vi "FPGA_8a_2ws_BIdireccional.vi"() -> ()   [LabVIEW 2015]
doc: "This VI reads a buffer of single point values from all four channels of the NI 923x and places the acquired data into a DMA FIFO."
uses:
  <vilib>/LabVIEW Targets/FPGA/cRIO/shared/nicrio_ModuleControls/nicrio_cRIO-9234_DataRatesRing2.ctl
  <vilib>/LabVIEW Targets/FPGA/cRIO/shared/nicrio_ModuleControls/nicrio_BasicConversionTime.ctl
  <vilib>/rvi/Emulation/niFpgaGetClockAttributes.vi
  <vilib>/rvi/Emulation/niFpgaSctlEmulationGetInTimedLoop.vi
  <vilib>/rvi/Emulation/niFpgaEmulationReportErrorSimple.vi
  <vilib>/rvi/Emulation/niFpgaProcessEmulError.vi
  <vilib>/rvi/eio/common/nirviEmuTemplateMethod_errors.vi
  <vilib>/rvi/Emulation/niFpgaCriticalErrorInLSC.vi
  <vilib>/rvi/eio/common/nirviEmuTemplatePropertySet_errors.vi
  <vilib>/rvi/interface/RandomDataEmulation/niFpgaRandomDataHandleErrors.vi
  <vilib>/eio/EIONode/EIONode.xnode
  <vilib>/eio/EIOPropertyNode/EIOPropertyNode.xnode
  <vilib>/rvi/DataTransferAndStorage/Container/XNode/niFpgaContainer.xnode
  <vilib>/rvi/interface/RandomDataEmulation/nirviRandomDataFpgaReadWriteTemplate.vi
  <vilib>/rvi/eio/common/nirviEmuTemplatePropertyGet_errors.vi
  <vilib>/rvi/eio/common/nirviEmuTemplatePropertyGet_noerrors.vi
  <vilib>/rvi/eio/common/nirviEmuTemplatePropertySet_noerrors.vi
panel:
  in  "Cycles to Filter":u16=5
  in  "Offset_WS2":fxp<+/-,24,-4>=0.000999998301267624 format="%.27g"
  in  "Canal cero WS2?":bool=TRUE
  out "NºRuedas 2":i32
  out "Nº Ruedas 1":i32
  out "Parar":bool
  out "RuedaDetectada2?":bool
  out "RuedaDetectada1?":bool
  out "Rueda2?":i16
  out "WhlCnt2":fxp<+/-,24,-4> format="%.27g"
  out "Direccion 0?":bool
  in  "Digital?":bool=TRUE
  out "Numeric 2":i32
  out "WhlCnt1":fxp<+/-,24,-4> format="%.27g"
  in  "Offset_WS1":fxp<+/-,24,-4>=0.000999998301267624 format="%.27g"
  out "Rueda1?":i16
  in  "Conversion Time":T1
  in  "Canal cero WS1?":bool=TRUE
  in  "Count(mSec)":u32=2
  out "Chassis Temperature":i16
  out "Detector de\npresencia":bool
  in  "Fotocélula":bool
  out "DC OK":bool
  in  "Data Rate":T2=2 items=["51.200 kS/s (NI 9234)"=1, "25.600 kS/s (NI 9234)"=2, "17.067 kS/s (NI 9234)"=3, "12.800 kS/s (NI 9234)"=4, "10.240 kS/s (NI 9234)"=5, "8.533 kS/s (NI 9234)"=6, "7.314 kS/s (NI 9234)"=7, "6.400 kS/s (NI 9234)"=8, "5.689 kS/s (NI 9234)"=9, "5.120 kS/s (NI 9234)"=10, "4.654 kS/s (NI 9234)"=11, "4.267 kS/s (NI 9234)"=12, "3.938 kS/s (NI 9234)"=13, "3.657 kS/s (NI 9234)"=14, "3.413 kS/s (NI 9234)"=15, "3.200 kS/s (NI 9234)"=16, "3.012 kS/s (NI 9234)"=17, "2.845 kS/s (NI 9234)"=18, "2.695 kS/s (NI 9234)"=19, "2.560 kS/s (NI 9234)"=20, "2.438 kS/s (NI 9234)"=21, "2.328 kS/s (NI 9234)"=22, "2.226 kS/s (NI 9234)"=23, "2.133 kS/s (NI 9234)"=24, "2.048 kS/s (NI 9234)"=25, "1.969 kS/s (NI 9234)"=26, "1.896 kS/s (NI 9234)"=27, "1.829 kS/s (NI 9234)"=28, "1.765 kS/s (NI 9234)"=29, "1.707 kS/s (NI 9234)"=30, "1.652 kS/s (NI 9234)"=31]
  out "Buffer Overflow":bool
  in  "Stop":bool
  out "Buffer Underflow":bool
  out "Error Out":errorcluster
  # "For instructions, and select Help>>Show Context Help and hover over the icon."
  # "Timing Parameters"
  # "Output Parameters"
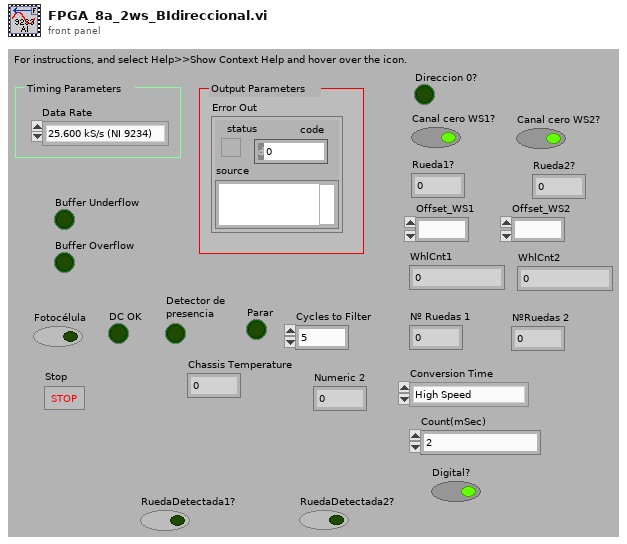
[diagram p1: front panel]
types:
  T1 = typedef "nicrio_BasicConversionTime.ctl" = enum8{"High Speed", "High Resolution"}
  T2 = typedef "nicrio_cRIO-9234_DataRatesRing2.ctl" = u8
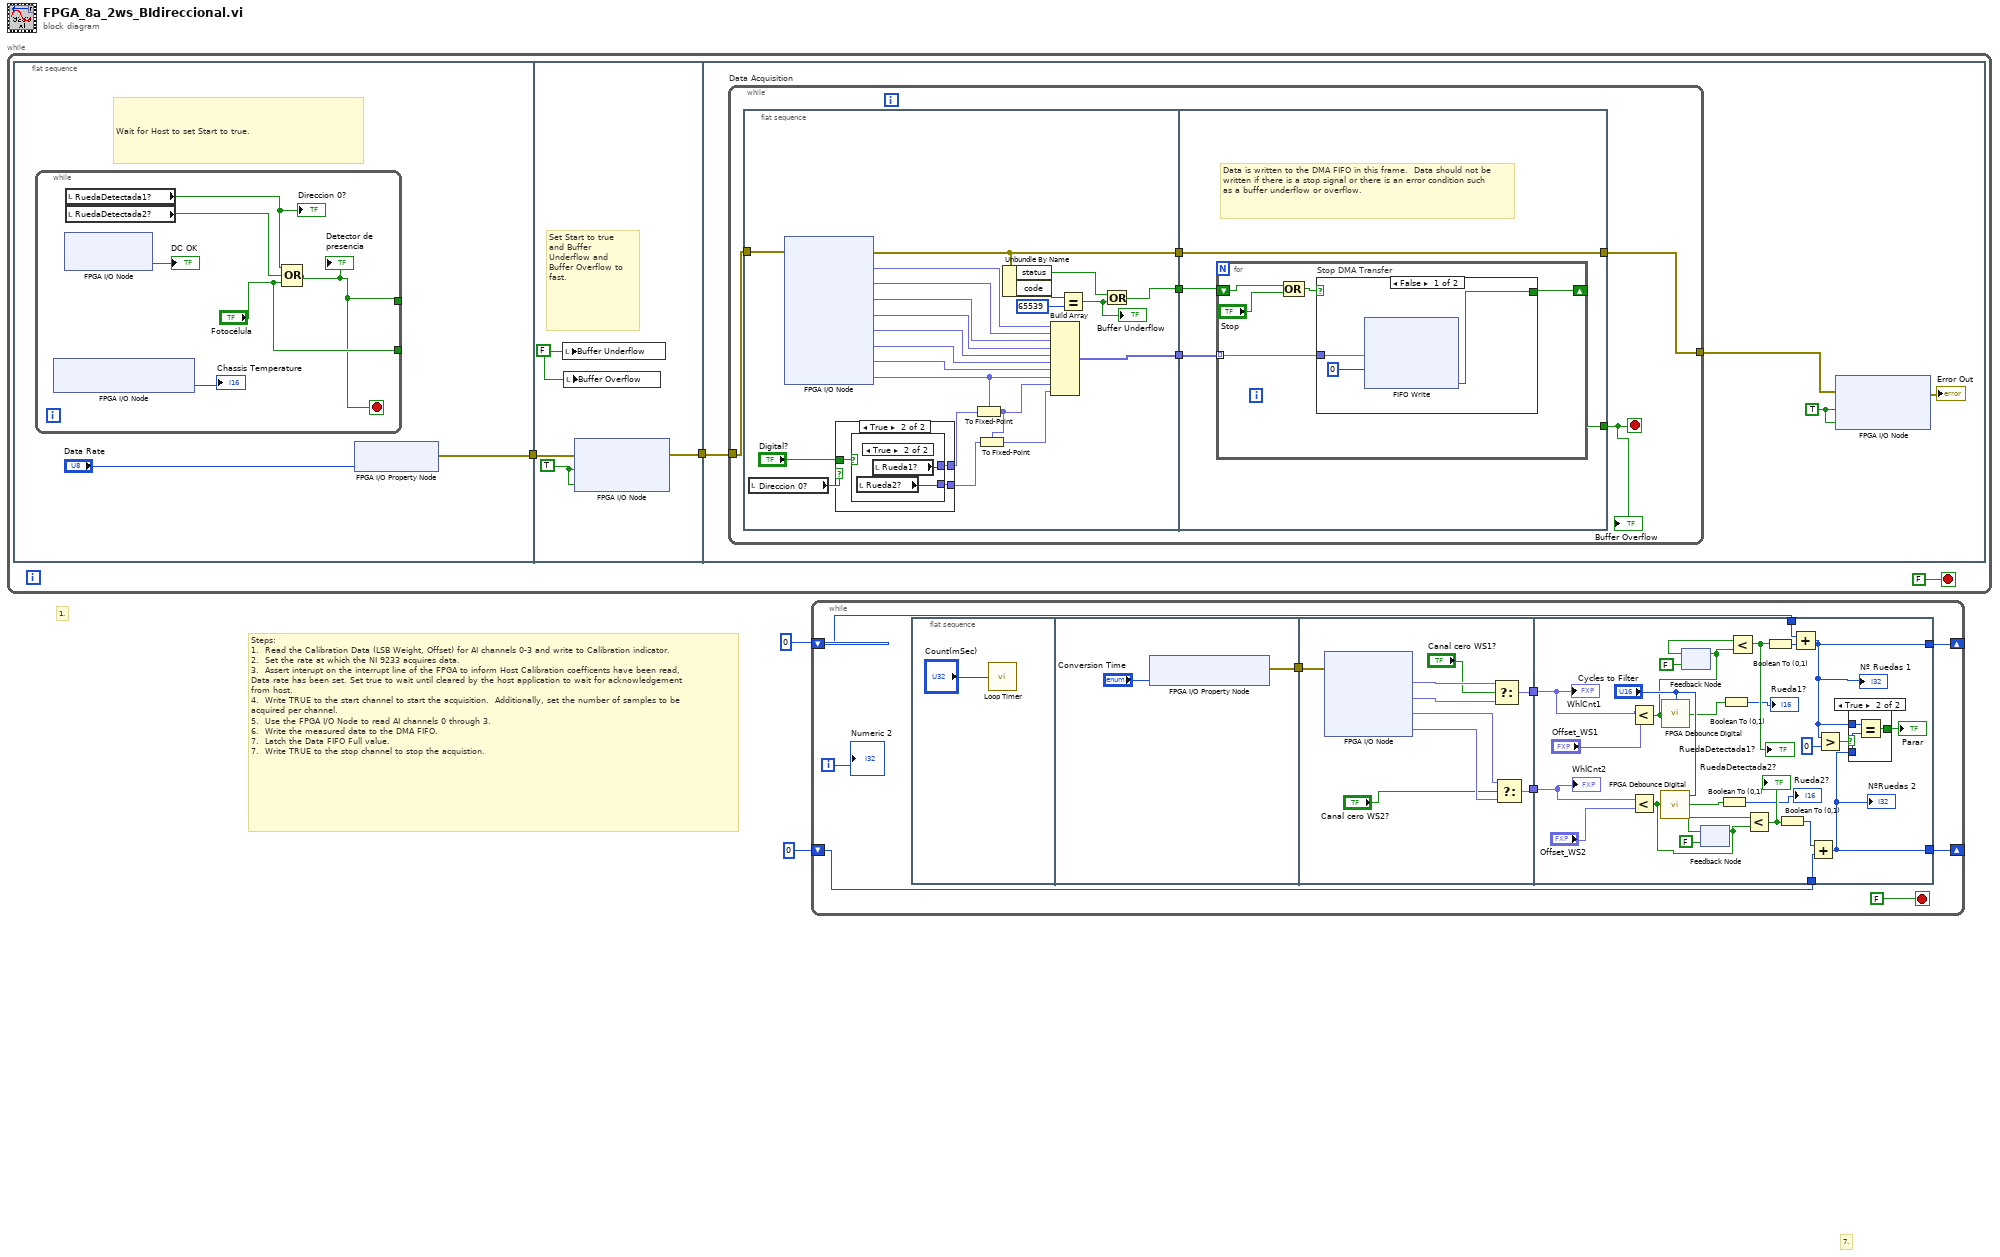
[diagram p0: block diagram]
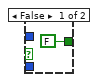
[diagram p2: hidden frame]
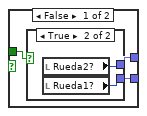
[diagram p3: hidden frame]
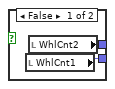
[diagram p4: hidden frame]
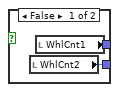
[diagram p5: hidden frame]
diagram:
  # "Steps: \n1.  Read the Calibration Data (LSB Weight, Offset) for AI channels 0-3 and write to Calibration indicator.\n2.  Set the rate at which the NI 9233 acquires data. \n3.  Assert interupt on the interrupt line of the FPGA to inform Host Calibration coefficents have been read, Data rate has been set. Set true to wait until cleared by the host application to wait for acknowledgement from host.\n4.  Write TRUE to the start channel to start the acquisition.  Additionally, set the number of samples to be acquired per channel.\n5.  Use the FPGA I/O Node to read AI channels 0 through 3. \n6.  Write the measured data to the DMA FIFO.\n7.  Latch the Data FIFO Full value.\n7.  Write TRUE to the stop channel to stop the acquistion."
  # "1."
  # "7."
  n1 = while {
    stop <- FALSE stop-if-true
    n2 = flat-sequence "MainSeq" {
      tunnel: [w7] -> w4
      tunnel: w4 -> [w16]
      tunnel: [w15] -> w3
      tunnel: w3 -> [w21]
      frame #0 {
        # "Wait for Host to set Start to true."
        n3 = while "initWait" {
          tunnel: ["Fotocélula"] -> _
          tunnel: [w9] -> _
          stop <- w9 stop-if-true
          n4 = xnode "FPGA I/O Node"() -> ("Chassis Temperature"=→"Chassis Temperature":i16)  [unwired: 1 in, 1 out]
          n5 = xnode "FPGA I/O Node"() -> ("Mod3/DI2"=→"DC OK":bool)  [unwired: 2 in, 2 out]
          n6 = local read "RuedaDetectada1?"() -> (w8:bool)
          "Direccion 0?" <- w8
          n7 = local read "RuedaDetectada2?"() -> (w10:bool)
          n8 = Compound Arithmetic op=OR(w8, w10, "Fotocélula") -> (w9:bool)
          "Detector de\npresencia" <- w9
        }
        n9 = xnode "FPGA I/O Property Node"("Data Rate"="Data Rate") -> ("error out"=w7:errorcluster)  [unwired: 2 in, 1 out]
      }
      frame #1 {
        w14 = TRUE
        w17 = FALSE ("Late? (Latched)")
        # "Set Start to true and Buffer Underflow and Buffer Overflow to fast."
        n10 = local write "Buffer Underflow"(w17) -> ()
        n11 = local write "Buffer Overflow"(w17) -> ()
        n12 = xnode "FPGA I/O Node"("error in"=w16, "Mod1/Start"=w14, "Mod2/Start"=w14) -> ("error out"=w15:errorcluster)  [unwired: 2 in, 2 out]
      }
      frame #2 {
        w18 = TRUE
        n13 = while "Data Acquisition" {
          tunnel: w21 -> [w25]
          tunnel: [w24] -> w19
          stop <- w22 stop-if-true
          n14 = flat-sequence "Data Acquisition Sequence" {
            tunnel: [w48] -> w27
            tunnel: [w39] -> w26
            tunnel: w25 -> [w47]
            tunnel: [w46] -> w23
            tunnel: w27 -> [w67]
            tunnel: w26 -> [w66]
            tunnel: [w65] -> w22
            tunnel: [w64] -> w24
            tunnel: w23 -> [w64]
            frame #0 {
              n15 = local read "Direccion 0?"() -> (w31:bool)
              n16 = xnode "FPGA I/O Node"("error in"=w47) -> ("error out"=w46:errorcluster, "Mod1/AI0"=w49:fxp<+/-,24,4>, "Mod1/AI1"=w42:fxp<+/-,24,4>, "Mod1/AI2"=w41:fxp<+/-,24,4>, "Mod1/AI3"=w40:fxp<+/-,24,4>, "Mod2/AI0"=w37:fxp<+/-,24,4>, "Mod2/AI1"=w36:fxp<+/-,24,4>, "Mod2/AI2"=w35:fxp<+/-,24,4>, "Mod2/AI3"=w34:fxp<+/-,24,4>)  [unwired: 8 in, 8 out]
              n17 = case shown="True" w31 {
                tunnel: "Digital?" -> [w52 w59]
                tunnel: [w51 w58] -> w33
                tunnel: [w50 w57] -> w30
                frame False {
                  n18 = case shown="True" w52 {
                    tunnel: [w54 w56] -> w51
                    tunnel: [w53 w55] -> w50
                    frame False {
                      n19 = local read "WhlCnt1"() -> (w53:fxp<+/-,24,-4>)
                      n20 = local read "WhlCnt2"() -> (w54:fxp<+/-,24,-4>)
                    }
                    frame True {
                      n21 = local read "Rueda2?"() -> (w56:i16)
                      n22 = local read "Rueda1?"() -> (w55:i16)
                    }
                  }
                }
                frame True {
                  n23 = case shown="True" w59 {
                    tunnel: [w61 w63] -> w58
                    tunnel: [w60 w62] -> w57
                    frame False {
                      n24 = local read "WhlCnt2"() -> (w60:fxp<+/-,24,-4>)
                      n25 = local read "WhlCnt1"() -> (w61:fxp<+/-,24,-4>)
                    }
                    frame True {
                      n26 = local read "Rueda2?"() -> (w62:i16)
                      n27 = local read "Rueda1?"() -> (w63:i16)
                    }
                  }
                }
              }
              n28 = To Fixed-Point(fixed-point type=w34, number=w33) -> (fixed-point=w29:fxp<+/-,24,4>)
              n29 = To Fixed-Point(fixed-point type=w29, number=w30) -> (fixed-point=w28:fxp<+/-,24,4>)
              n30 = Unbundle By Name(w46) -> ("status"=w38:bool, "code"=w45:i32)
              n31 = Build Array(w49, w42, w41, w40, w37, w36, w35, w34, w29, w28) -> (w48:fxp<+/-,24,4>[])
              n32 = Equal?(x=w45, y=65539) -> (x = y?=w43:bool)
              "Buffer Underflow" <- w43
              n33 = Or(x=w38, y=w43) -> (x .or. y?=w39:bool)
            }
            frame #1 {
              # "Data is written to the DMA FIFO in this frame.  Data should not be written if there is a stop signal or there is an error condition such as a buffer underflow or overflow."
              n34 = for "DMAWriteLoop" {
                tunnel: w67 -> [w72] mode=indexing
                shift-right: [w71] -> w65
                shift-left: w66 -> [w70]
                n35 = Compound Arithmetic op=OR(w70, "Stop") -> (w69:bool)
                n36 = case "Stop DMA Transfer" shown="False" w69 {
                  selector: w69 -> [_ w76]
                  tunnel: w72 -> [w73 _]
                  tunnel: [w75 w76] -> w71
                  frame False {
                    n37 = xnode ("FIFO Write")("Element"=w73, "Timeout"=0) -> ("Timed Out?"=w75:bool)  [unwired: 1 in, 1 out]
                  }
                  frame True {
                  }
                }
              }
            }
          }
          "Buffer Overflow" <- w22
        }
        n38 = xnode "FPGA I/O Node"("error in"=w19, "Mod1/Stop"=w18, "Mod2/Stop"=w18) -> ("error out"=→"Error Out":errorcluster)  [unwired: 2 in, 2 out]
      }
    }
  }
  n39 = while {
    shift-right: [w82] -> _
    shift-left: 0 -> [w81]
    shift-right: [w79] -> _
    shift-left: 0 -> [w80]
    i -> [w78]
    stop <- FALSE stop-if-true
    n40 = flat-sequence {
      tunnel: [w87] -> w84
      tunnel: [w97] -> w85
      tunnel: w84 -> [w91]
      tunnel: [w94] -> w83
      tunnel: w85 -> [w123]
      tunnel: w83 -> [w121]
      tunnel: [w111] -> w82
      tunnel: w81 -> [w118]
      tunnel: w80 -> [w116]
      tunnel: [w110] -> w79
      frame #0 {
        n41 = call "Loop Timer"("Count(mSec)"="Count(mSec)") -> ()  [unwired: 1 out]
      }
      frame #1 {
        n42 = xnode "FPGA I/O Property Node"("Conversion Time"="Conversion Time") -> ("error out"=w87:errorcluster)  [unwired: 2 in, 1 out]
      }
      frame #2 {
        n43 = xnode "FPGA I/O Node"("error in"=w91) -> ("Mod4/AI0"=w96:fxp<+/-,24,-4>, "Mod4/AI1"=w95:fxp<+/-,24,-4>, "Mod4/AI2"=w93:fxp<+/-,24,-4>, "Mod4/AI3"=w92:fxp<+/-,24,-4>)  [unwired: 4 in, 5 out]
        n44 = Select(t=w96, s="Canal cero WS1?", f=w95) -> (s? t:f=w97:fxp<+/-,24,-4>)
        n45 = Select(t=w93, s="Canal cero WS2?", f=w92) -> (s? t:f=w94:fxp<+/-,24,-4>)
      }
      frame #3 {
        n46 = Less?(x=w123, y="Offset_WS1") -> (x < y?=w101:bool)
        n47 = Less?(x=w121, y="Offset_WS2") -> (x < y?=w99:bool)
        n48 = call "FPGA Debounce Digital.vi"("Input Signal"=w99, "Cycles to Filter"="Cycles to Filter") -> ("Output Filtered Signal"=w98:bool)
        n49 = call "FPGA Debounce Digital.vi"("Input Signal"=w101, "Cycles to Filter"="Cycles to Filter") -> ("Output Filtered Signal"=w100:bool)
        n50 = feedback-in #1(w101) -> ()
        n51 = feedback #1(FALSE) -> (w119:bool)
        n52 = feedback #2(FALSE) -> (w112:bool)
        n53 = feedback-in #2(w99) -> ()
        n54 = Boolean To (0,1)(Boolean=w98) -> (0, 1=→"Rueda2?":i16)
        n55 = Boolean To (0,1)(Boolean=w100) -> (0, 1=→"Rueda1?":i16)
        n56 = Less?(x=w119, y=w101) -> (x < y?=w107:bool)
        "RuedaDetectada1?" <- w107
        n57 = Less?(x=w112, y=w99) -> (x < y?=w106:bool)
        "RuedaDetectada2?" <- w106
        n58 = Boolean To (0,1)(Boolean=w107) -> (0, 1=w103:i16)
        n59 = Boolean To (0,1)(Boolean=w106) -> (0, 1=w108:i16)
        n60 = Add(x=w118, y=w103) -> (x+y=w111:i32)
        "Nº Ruedas 1" <- w111
        n61 = Add(x=w108, y=w116) -> (x+y=w110:i32)
        "NºRuedas 2" <- w110
        n62 = Greater?(x=w111, y=i64 0) -> (0:w113:bool)
        n63 = case shown="True" w113 {
          tunnel: w110 -> [_ w127]
          tunnel: w111 -> [_ w126]
          tunnel: [FALSE w125] -> w115
          frame False {
          }
          frame True {
            n64 = Equal?(x=w126, y=w127) -> (x = y?=w125:bool)
          }
        }
        "Parar" <- w115
        "WhlCnt1" <- w123
        "WhlCnt2" <- w121
      }
    }
    "Numeric 2" <- w78
  }
